vi "Main.vi"(11 "Module Admin":refnum<class "Delacor_lib_QMH_Cloneable Module Admin.lvclass">) -> ()   [LabVIEW 2020, in "DQMH module.lvlib"]
doc: "This template is based off of the Queued Message Handler design pattern and the Queued Message Handler project template that ships with LabVIEW.\n\nThe main difference is that the queue is private to this module and communication between modules is performed via Broadcast and Request events.\n\nRequest events are wrapped in public API methods and are handled in the Event Handling Loop (EHL) of this VI. Any module can register for Broadcast events sent by this module. The EHL generates messages based on user interface actions.\n\nThe Message Handling Loop (MHL) processes messages generated by the EHL, or by other messages. The messages are string values, so new messages can be added easily to the Message Cases case structure in the MHL. Each message cluster can also provide an optional value for Message Data, which is a variant that can be converted to whatever message-specific data is required.\n_____\nBased on Delacor QMH Project Template 5.0.0.82."
uses:
  DQMH module.lvlib
  <vilib>/Delacor/Delacor QMH/Libraries/Cloneable Module Admin_class/Delacor_lib_QMH_Cloneable Module Admin.lvclass
  C:/Program Files (x86)/National Instruments/LabVIEW 2020/vi.lib/Delacor/Delacor QMH/Libraries/Module Admin_class/Delacor_lib_QMH_Module Admin.lvclass
  implementations/Combo box/serial device brand.ctl
  Module Data--cluster.ctl
  <vilib>/Delacor/Delacor QMH/Libraries/Cloneable Module Admin_class/Delacor_lib_QMH_Cloneable Module Admin.lvclass/Delacor_lib_QMH_Cloneable Module Admin.ctl
  Stop Argument--cluster.ctl
  <vilib>/Delacor/Delacor QMH/Libraries/Message Queue_class/Delacor_lib_QMH_Message Queue.lvclass/Delacor_lib_QMH_Message Queue.ctl
  <vilib>/Delacor/Delacor QMH/Libraries/Module Admin_class/Delacor_lib_QMH_Module Admin.lvclass/Delacor_lib_QMH_Module Admin.ctl
  Read ADC Argument--cluster.ctl
  Set Port Status Argument--cluster.ctl
  Get Port Status Argument--cluster.ctl
  Set Pin Argument--cluster.ctl
  Get Pin Status Argument--cluster.ctl
  <vilib>/Utility/miscctls.llb/LVPointTypeDef.ctl
  implementations/Arduino/Arduino.lvclass
  D:/fork/Hal-Proyecto-/Abstracts/Serial Device/Serial Device.lvclass
  Abstracts/Serial Device/Serial Device.lvclass
  implementations/Cypress/Cypress.lvclass
  implementations/Simulado/Simulado.lvclass
  <vilib>/Delacor/Delacor QMH/Libraries/Cloneable Module Admin_class/Delacor_lib_QMH_Get Module ID.vi
  <vilib>/Delacor/Delacor QMH/Libraries/Message Queue_class/Delacor_lib_QMH_Enqueue Message (Single).vi
  <vilib>/Delacor/Delacor QMH/Libraries/Module Admin_class/Delacor_lib_QMH_Get External Launch.vi
  <vilib>/Utility/error.llb/Error Cluster From Error Code.vi
  <vilib>/ErrorRing/Error Ring.xnode
  <vilib>/Delacor/Delacor QMH/Libraries/Message Queue_class/Delacor_lib_QMH_Message Queue.lvclass
panel:
  in  "Configurar":bool
  in  "VISA resource name":refnum<visa-resource-name>
  in  "Serial Device Brand":T1
  out "Respuesta":string
  in  "CH":dbl
  in  "Read ADC":bool
  in  "Value":string
  in  "Puerto":dbl
  in  "Set port":bool
  out "Port status":bool[](array[boolean])
  in  "Port":dbl
  in  "Get port":bool
  in  "Value":bool
  in  "Pin":dbl
  in  "Port 2":dbl
  in  "Set Pin":bool
  out "error out":errorcluster
  out "Value":bool
  in  "Pin 2":dbl
  in  "Port 3":dbl
  in  "Get pin":bool
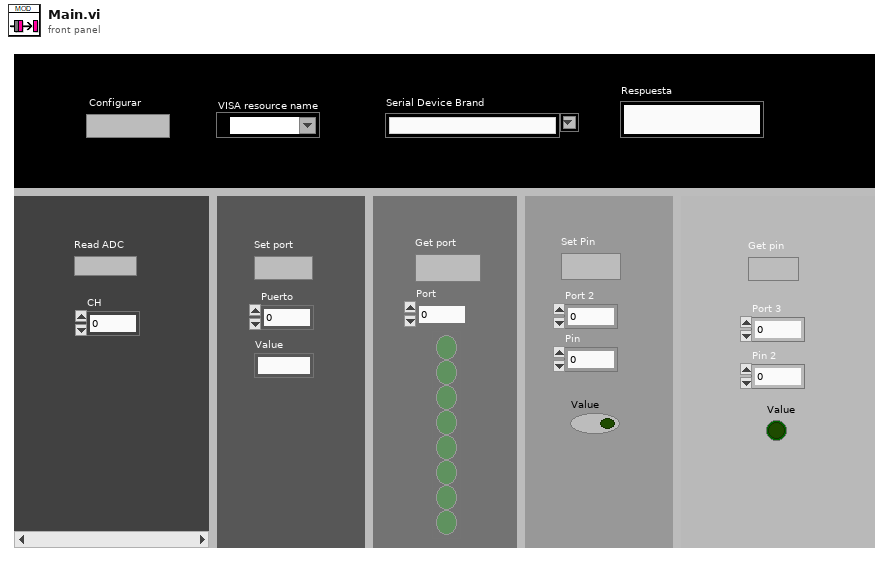
[diagram p1: front panel]
types:
  T1 = typedef "Serial Device.lvclass/serial device brand.ctl" = string
  T2 = typedef "DQMH module.lvlib/Request Events--cluster.ctl" = cluster{"Stop Module":refnum<user-event>, "Show Panel":refnum<user-event>, "Hide Panel":refnum<user-event>, "Show Diagram":refnum<user-event>, "Get Module Execution Status":refnum<user-event>, "Read ADC":refnum<user-event>, "Set Port Status":refnum<user-event>, "Get Port Status":refnum<user-event>, "Set Pin":refnum<user-event>, "Get Pin Status":refnum<user-event>}
  T3 = typedef "DQMH module.lvlib/Module Data--cluster.ctl" = cluster{"Status":string}
  T4 = enum32{"invalid lock state", "Not Locked", "Locked (No Password)", "Password-protected"}
  T5 = typedef "DQMH module.lvlib/Stop Argument--cluster.ctl" = cluster{"Module ID":i32, "Origin":string, "Exit via Stop Module Req?":bool, "Wait for Module to stop?":bool}
  T6 = typedef "DQMH module.lvlib/Read ADC Argument--cluster.ctl" = cluster{"Module ID":i32, "CH ADC":dbl}
  T7 = typedef "DQMH module.lvlib/Set Port Status Argument--cluster.ctl" = cluster{"Module ID":i32, "Puerto":dbl, "Value":string}
  T8 = typedef "DQMH module.lvlib/Get Port Status Argument--cluster.ctl" = cluster{"Module ID":i32, "Port":dbl}
  T9 = typedef "DQMH module.lvlib/Set Pin Argument--cluster.ctl" = cluster{"Module ID":i32, "Port":dbl, "Pin":dbl, "Value":bool}
  T10 = typedef "DQMH module.lvlib/Get Pin Status Argument--cluster.ctl" = cluster{"Module ID":i32, "Port":dbl, "Pin":dbl, "Valor de Pin":bool}
  T11 = enum32{"Invalid", "Standard", "Closed", "Hidden", "Minimized", "Maximized"}
  T12 = typedef "LVPointTypeDef.ctl" = cluster{"Horizontal":i16, "Vertical":i16}
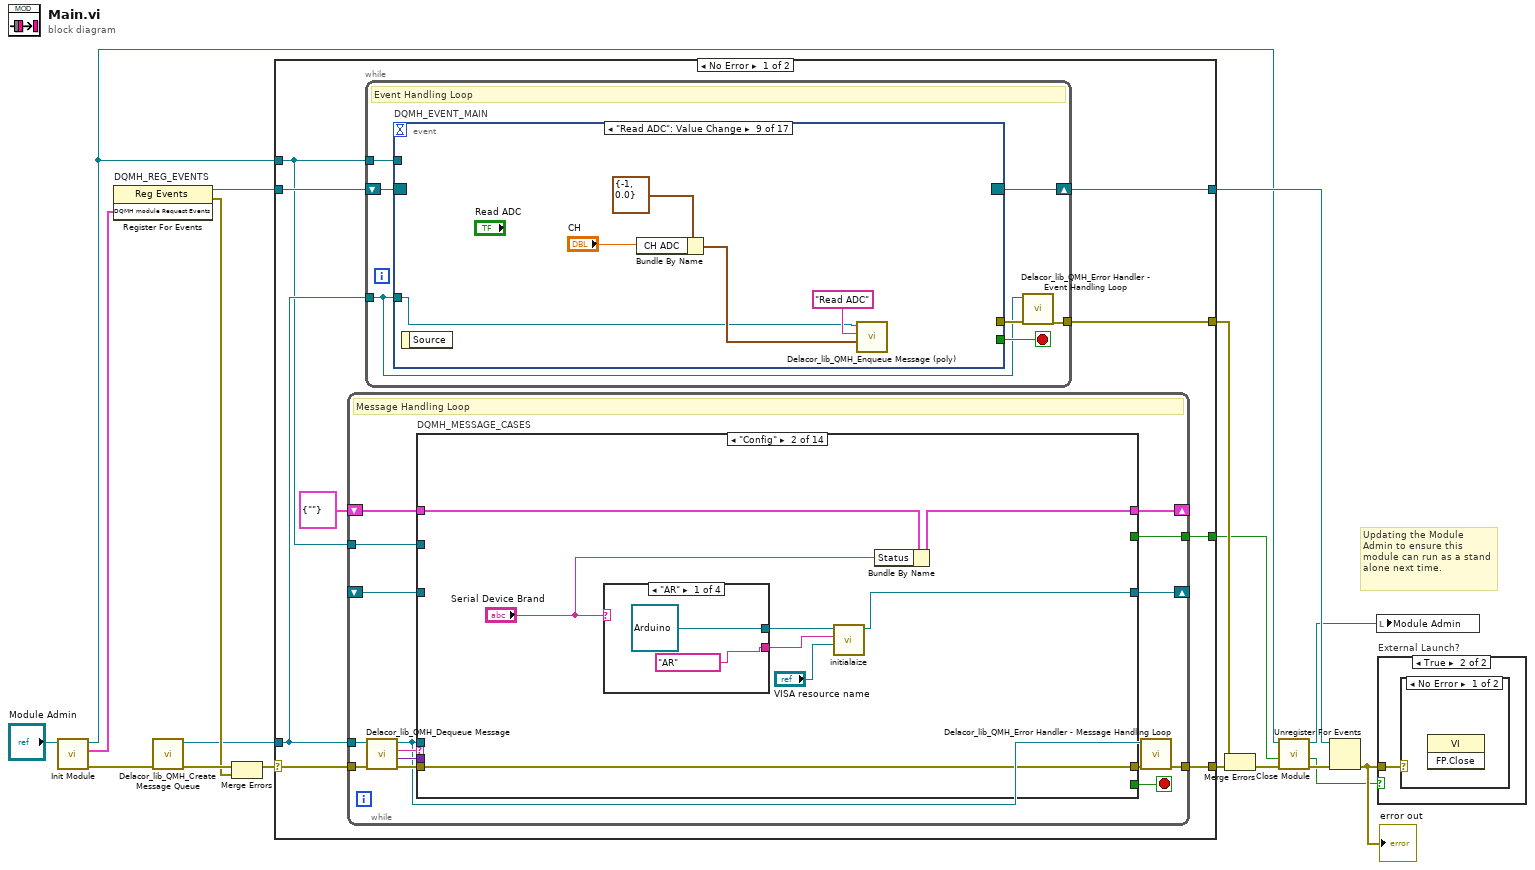
[diagram p0: block diagram]
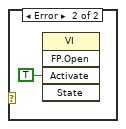
[diagram p3: hidden frame]
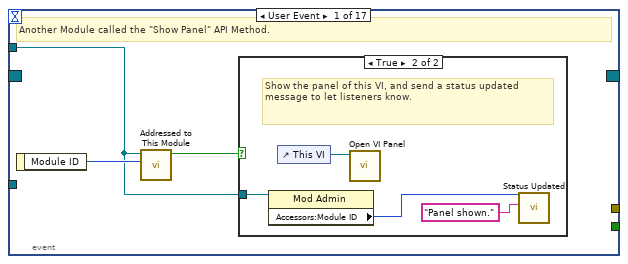
[diagram p4: hidden frame]
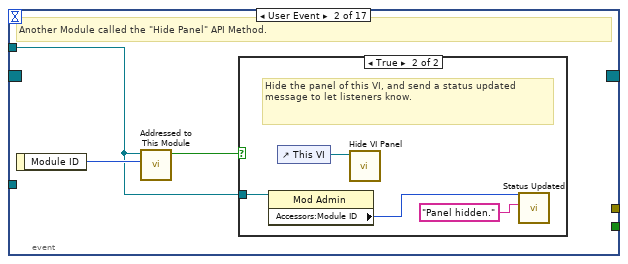
[diagram p6: hidden frame]
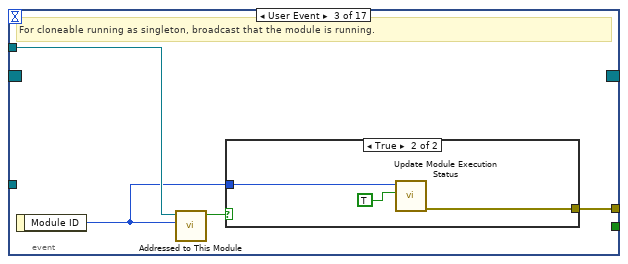
[diagram p8: hidden frame]
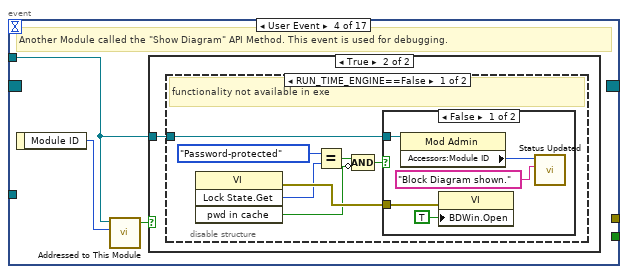
[diagram p10: hidden frame]
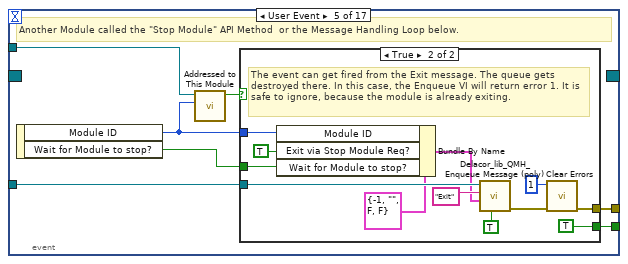
[diagram p14: hidden frame]
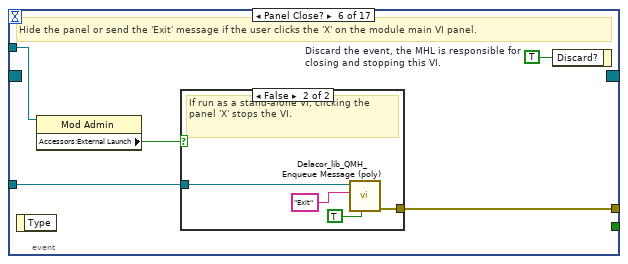
[diagram p16: hidden frame]
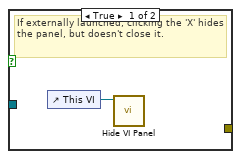
[diagram p17: hidden frame]
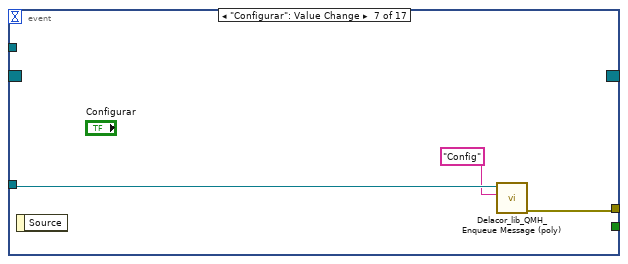
[diagram p18: hidden frame]
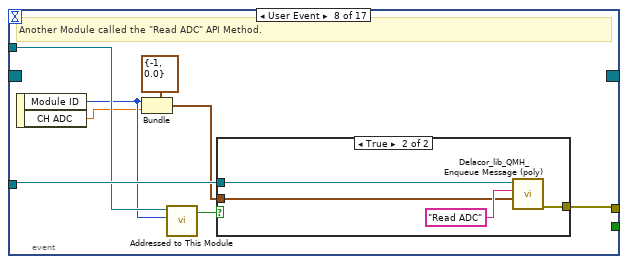
[diagram p19: hidden frame]
diagram:
  # "Updating the Module Admin to ensure this module can run as a stand alone next time."
  n1 = call "Init Module.vi"("Cloneable Module Admin in"="Module Admin") -> ("error out"=w15:errorcluster, "DQMH module Request Events"=w7:T2, "Cloneable Module Admin out"=w4:refnum<class "Delacor_lib_QMH_Cloneable Module Admin.lvclass">)  [unwired: 8 in]
  n2 = register-events "DQMH_REG_EVENTS"(w7) -> (reference out=w8:refnum<event-registration>, error out=w10:errorcluster)  [unwired: 2 in]
  n3 = call <vilib>:"Delacor_lib_QMH_Create Message Queue.vi"("error in (no error)"=w15) -> ("error out"=w12:errorcluster, "Message Queue"=w6:refnum<class "Delacor_lib_QMH_Message Queue.lvclass">)  [unwired: 9 in]
  n4 = Merge Errors(w12, w10) -> (w11:errorcluster)
  n5 = case shown="No Error" w11 {
    selector: w11 -> [w25 w417]
    tunnel: [w27 w416] -> w16
    tunnel: [w24 w424] -> w9
    tunnel: w8 -> [w22 w424]
    tunnel: w6 -> [w21 w415]
    tunnel: [w26 _] -> w17
    tunnel: w4 -> [w20 w420]
    tunnel: [w19 _] -> w2
    frame No Error {
      n6 = while {
        tunnel: w21 -> [w207]
        shift-right: [w211] -> _
        shift-left: T3 {"Status"=""} ("Data Cluster") -> [w212]
        tunnel: w25 -> [w215]
        tunnel: [w213] -> w27
        tunnel: w20 -> [w205]
        tunnel: [w204] -> w19
        shift-right: [w203] -> _
        shift-left: _ -> [w202]
        stop <- w210 stop-if-true
        # "Message Handling Loop"
        n7 = call-dynamic "Delacor_lib_QMH_Dequeue Message.vi"("error in (no error)"=w215, "Message Queue in"=w207) -> ("error out"=w214:errorcluster, "Message Data"=w208:variant, "Message"=w209:string, "Message Queue out"=w206:refnum<class "Delacor_lib_QMH_Message Queue.lvclass">)  [unwired: 6 in]
        n8 = case "DQMH_MESSAGE_CASES" shown="\"Config\"" w209 {
          selector: w209 -> [_ _ _ _ _ _ _ _ _ _ _ _ _ w402]
          tunnel: w206 -> [_ _ _ w256 _ w282 _ w320 _ _ _ w358 w391 _]
          tunnel: w214 -> [w233 w243 w254 w270 w275 w294 w310 w329 w346 w350 w353 w366 w397 w404]
          tunnel: [w231 w243 w254 w258 w276 w285 w300 w318 w334 w349 w353 w362 w394 w405] -> w216
          tunnel: w212 -> [w217 w238 w253 w269 w277 w293 w309 w328 w345 w348 w352 w356 w390 w403]
          tunnel: [w217 w239 w253 w269 w277 w293 w309 w328 w345 w348 w352 w356 w390 w403] -> w211
          tunnel: [_ _ _ _ _ _ _ _ _ _ _ _ w389 _] -> w210
          tunnel: w208 -> [_ _ _ w268 w274 w292 w308 w327 w344 _ _ w361 w387 _]
          tunnel: w205 -> [w220 _ _ _ _ _ _ _ _ _ _ w360 w383 w400]
          tunnel: [_ _ _ _ _ _ _ _ _ _ _ _ w385 _] -> w204
          tunnel: [w218 w236 w252 w255 w271 w280 w303 w321 w339 w347 w351 w354 w380 w398] -> w203
          tunnel: w202 -> [w218 _ w252 w265 w271 w289 w305 w323 w340 w347 w351 w354 w381 w398]
          frame "Initialize" {
            (unwired) T12 {"Horizontal"=0, "Vertical"=0} ("Origin")
            # "Initialize - Any operation that needs to be done before the module can receive messages. Synchronize Caller Events.vi will inform Start Module.vi that the module has launched and is ready to receive messages. Module Did Init.vi will broadcast that the module initialized."
            n9 = call "Synchronize Caller Events.vi"("error in (no error)"=w233, "Module Admin"=w220) -> ("error out"=w232:errorcluster, "Module Admin out"=w219:refnum<class "Delacor_lib_QMH_Cloneable Module Admin.lvclass">)  [unwired: 8 in]
            n10 = property class="Mod Admin"(reference=w219) -> ("Accessors:Module ID"=w222:i32, "Accessors:External Launch"=w221:bool)  [unwired: 1 in, 2 out]
            n11 = call "Module Name--constant.vi"("Module ID"=w222) -> ("Module Name"=w228:string)  [unwired: 10 in]
            n12 = property class="VI"("Front Panel.Title"=w228) -> (reference out=w230:refnum<vi>, error out=w235:errorcluster)  [unwired: 2 in]
            n13 = Select(t=T11."Hidden" ("State"), s=w221, f=T11."Standard" ("State")) -> (s? t:f=w225:T11)
            n14 = invoke class="VI" method="FP.Open"(reference=w230, error in=w235, "State"=w225) -> (reference out=w229:refnum<vi>, error out=w234:errorcluster)  [unwired: 2 in, 3 out]
            n15 = call "Module Name--constant.vi"("Module ID"=w222) -> ("Module Name"=w223:string)  [unwired: 10 in]
            n16 = invoke class="VI" method="FP.Center"(reference=w229, error in=w234) -> ()  [unwired: 1 in, 3 out]
            n17 = call "Module Did Init.vi"("error in (no error)"=w232, "Initialized?"=TRUE, "Origin"=w223, "Module ID"=w222) -> ("error out"=w231:errorcluster)  [unwired: 7 in]
          }
          frame "Config" {
            n18 = case shown="\"AR\"" "Serial Device Brand" {
              tunnel: [refnum<class "Arduino.lvclass"> refnum ("Arduino.lvclass") refnum<class "Serial Device.lvclass"> refnum ("Cypress.lvclass") refnum<class "Cypress.lvclass"> refnum ("Cypress.lvclass") refnum<class "Simulado.lvclass"> refnum ("Simulado.lvclass")] -> w242
              tunnel: [T1 "AR" ("Serial Device Brand 2") T1 "NX" ("Serial Device Brand 2") T1 "CY" ("Serial Device Brand 2") T1 "SD" ("Serial Device Brand 2")] -> w240
              frame "AR" {
              }
              frame "NX" {
              }
              frame "CY" {
              }
              frame "SD", Default {
              }
            }
            n19 = call-dynamic "initialaize.vi"("Visa com port"="VISA resource name", "Serial Device Brand"=w240, "Serial Device in"=w242) -> ("Serial Device out"=w236:refnum<class "Serial Device.lvclass">)  [unwired: 7 in, 1 out]
            n20 = Bundle By Name(cluster=w238, "Status"="Serial Device Brand") -> (w239:T3)
          }
          frame "--- Module Specific ---" {
            # "Separator -- The following cases handle messages specific to this Module."
          }
          frame "Read ADC" {
            n21 = Variant To Data(error in=w270, type=T6 {"Module ID"=-1, "CH ADC"=0.0} ("Read ADC Argument"), Variant=w268) -> (data=w266:T6, error out=w259:errorcluster)
            n22 = Unbundle By Name(w266) -> ("CH ADC"=w263:dbl)
            n23 = call-dynamic "Read ADC.vi"("ADC CH"=w263, "Serial Device in"=w265) -> ("error out"=w262:errorcluster, "Serial Device out"=w264:refnum<class "Serial Device.lvclass">)  [unwired: 8 in]
            n24 = call-dynamic "Read Response ADC.vi"("error in (no error)"=w262, "Serial Device in"=w264) -> ("Respuesta"=w261:string, "Serial Device out"=w255:refnum<class "Serial Device.lvclass">)  [unwired: 7 in, 1 out]
            n25 = call-poly <vilib>:"Delacor_lib_QMH_Enqueue Message (poly).vi"("Message Data"=w261, "Message"="Response", "Message Queue in"=w256) -> ("error out"=w257:errorcluster)  [unwired: 7 in, 1 out]
            n26 = Merge Errors(w257, w259) -> (w258:errorcluster)
          }
          frame "Response" {
            n27 = Variant To Data(error in=w275, type="", Variant=w274) -> (data=→"Respuesta":string, error out=w276:errorcluster)
          }
          frame "Set Port Status" {
            n28 = Variant To Data(error in=w294, type=T7 {"Module ID"=-1, "Puerto"=0.0, "Value"=""} ("Set Port Status Argument"), Variant=w292) -> (data=w290:T7, error out=w286:errorcluster)
            n29 = Unbundle By Name(w290) -> ("Puerto"=w279:dbl, "Value"=w278:string)
            n30 = call-dynamic "Set port.vi"("Value"=w278, "Puerto"=w279, "Serial Device in"=w289) -> ("error out"=w287:errorcluster, "Serial Device out"=w288:refnum<class "Serial Device.lvclass">)  [unwired: 7 in]
            n31 = call-dynamic "Read Response ADC.vi"("error in (no error)"=w287, "Serial Device in"=w288) -> ("Respuesta"=w281:string, "Serial Device out"=w280:refnum<class "Serial Device.lvclass">)  [unwired: 7 in, 1 out]
            n32 = call-poly <vilib>:"Delacor_lib_QMH_Enqueue Message (poly).vi"("Message Data"=w281, "Message"="Response", "Message Queue in"=w282) -> ("error out"=w284:errorcluster)  [unwired: 7 in, 1 out]
            n33 = Merge Errors(w284, w286) -> (w285:errorcluster)
          }
          frame "Get Port Status" {
            n34 = Variant To Data(error in=w310, type=T8 {"Module ID"=-1, "Port"=0.0} ("Get Port Status Argument"), Variant=w308) -> (data=w306:T8, error out=w299:errorcluster)
            n35 = Unbundle By Name(w306) -> ("Port"=w302:dbl)
            n36 = call-dynamic "Get port Status.vi"("Puerto"=w302, "Serial Device in"=w305) -> ("error out"=w298:errorcluster, "Serial Device out"=w304:refnum<class "Serial Device.lvclass">)  [unwired: 8 in]
            n37 = call-dynamic "Get status Response.vi"("error in (no error)"=w298, "Serial Device in"=w304) -> ("error out"=w297:errorcluster, "Response"=w301:string, "Serial Device out"=w303:refnum<class "Serial Device.lvclass">)  [unwired: 7 in]
            n38 = Hexadecimal String To Number(string=w301) -> (number=w296:u32)  [unwired: 2 in, 1 out]
            n39 = Number To Boolean Array(number=w296) -> (Boolean array=→"Port status":bool[])
            n40 = Merge Errors(w297, w299) -> (w300:errorcluster)
          }
          frame "Set Pin" {
            n41 = Variant To Data(error in=w329, type=T9 {"Module ID"=-1, "Port"=0.0, "Pin"=0.0, "Value"=FALSE} ("Set Pin Argument"), Variant=w327) -> (data=w325:T9, error out=w319:errorcluster)
            n42 = Unbundle By Name(w325) -> ("Port"=w314:dbl, "Pin"=w313:dbl, "Value"=w312:bool)
            n43 = call-dynamic "Set pin status.vi"("Value"=w312, "Pin"=w313, "Port"=w314, "Serial Device in"=w323) -> ("error out"=w324:errorcluster, "Serial Device out"=w322:refnum<class "Serial Device.lvclass">)  [unwired: 6 in]
            n44 = call-dynamic "Read Response ADC.vi"("error in (no error)"=w324, "Serial Device in"=w322) -> ("error out"=w315:errorcluster, "Respuesta"=w311:string, "Serial Device out"=w321:refnum<class "Serial Device.lvclass">)  [unwired: 7 in]
            n45 = call-poly <vilib>:"Delacor_lib_QMH_Enqueue Message (poly).vi"("error in (no error)"=w315, "Message Data"=w311, "Message"="Response", "Message Queue in"=w320) -> ("error out"=w317:errorcluster)  [unwired: 6 in, 1 out]
            n46 = Merge Errors(w317, w319) -> (w318:errorcluster)
          }
          frame "Get Pin Status" {
            n47 = Variant To Data(error in=w346, type=T10 {"Module ID"=-1, "Port"=0.0, "Pin"=0.0, "Valor de Pin"=FALSE} ("Get Pin Status Argument"), Variant=w344) -> (data=w342:T10, error out=w335:errorcluster)
            n48 = Unbundle By Name(w342) -> ("Port"=w337:dbl, "Pin"=w336:dbl)
            n49 = call-dynamic "Get pin Status.vi"("Pin 2"=w336, "Puerto"=w337, "Serial Device in"=w340) -> ("error out"=w338:errorcluster, "Serial Device out"=w341:refnum<class "Serial Device.lvclass">)  [unwired: 7 in]
            n50 = call-dynamic "Get pin Status Response.vi"("error in (no error)"=w338, "Serial Device in"=w341) -> ("Value"=w333:string, "Serial Device out"=w339:refnum<class "Serial Device.lvclass">)  [unwired: 7 in, 1 out]
            n51 = Hexadecimal String To Number(string=w333) -> (number=w332:u32)  [unwired: 2 in, 1 out]
            n52 = Equal To 0?(x=w332) -> (x = 0?=w331:bool)
            n53 = Not(x=w331) -> (.not. x?=→"Value":bool)
            n54 = Merge Errors(w335) -> (w334:errorcluster)
          }
          frame "---Copy This Frame---" {
            # "Duplicate this frame when creating new messages.  Change this comment in the duplicated frame to describe this message."
            n55 = Merge Errors(w350) -> (w349:errorcluster)
          }
          frame "--- Exit and Error Handling---" {
            # "Separator - the following cases handle errors and exit messages."
          }
          frame "Error" {
            # "Error - Check the error message data and respond accordingly. This message is sent by the \"Error Handler\" VIs at the end of each loop in this application."
            n56 = property class="Mod Admin"(reference=w360) -> ("Accessors:External Launch"=w359:bool, "Accessors:Module ID"=w357:i32)  [unwired: 1 in, 2 out]
            n57 = Variant To Data(error in=w366, type=errorcluster {"status"=FALSE, "code"=0, "source"=""} ("error constant"), Variant=w361) -> (data=w367:errorcluster, error out=w364:errorcluster)
            n58 = Unbundle By Name(w356) -> ("Status"=w355:string)
            n59 = call "Module Name--constant.vi"("Module ID"=w357) -> ()  [unwired: 10 in, 1 out]
            n60 = case shown="True" w359 {
              tunnel: [w372 w374] -> w363
              tunnel: w358 -> [w370 w376]
              tunnel: w367 -> [w371 _]
              tunnel: w355 -> [_ w379]
              frame False {
                n61 = call <vilib>:"Simple Error Handler.vi"("error in (no error)"=w371) -> ()  [unwired: 4 in, 5 out]
                n62 = call-poly <vilib>:"Delacor_lib_QMH_Enqueue Message (poly).vi"("Priority Message? (F)"=TRUE, "Message"="Exit", "Message Queue in"=w370) -> ("error out"=w372:errorcluster)  [unwired: 7 in, 1 out]
              }
              frame True {
                n63 = Concatenate Strings("Micro desconectado" ("string"), w379) -> (w377:string)
                n64 = call-poly <vilib>:"Delacor_lib_QMH_Enqueue Message (poly).vi"("Priority Message? (F)"=TRUE, "Message"="EXIT", "Message Queue in"=w376) -> ("error out"=w374:errorcluster)  [unwired: 7 in, 1 out]
                n65 = One Button Dialog(message=w377) -> ()  [unwired: 1 in, 1 out]
              }
            }
            n66 = call "Error Reported.vi"("Additional Information"=w355, "Error"=w367, "Module ID"=w357) -> ()  [unwired: 8 in, 1 out]
            n67 = Merge Errors(w364, w363) -> (w362:errorcluster)
            n68 = local write "error out"(w362) -> ()
          }
          frame "Exit" {
            w388 = 91  # 91: not all Exit messages will have an argument
            w389 = TRUE  # Stop the VI
            # "Release the message queue reference"
            # "Exit - Exit the application."
            n69 = Variant To Data(error in=w397, type=T5 {"Module ID"=-1, "Origin"="", "Exit via Stop Module Req?"=FALSE, "Wait for Module to stop?"=FALSE} ("Stop Argument"), Variant=w387) -> (data=w384:T5, error out=w392:errorcluster)
            n70 = call <vilib>:"Clear Errors.vi"("error in (no error)"=w392, "specific error code to clear (0: all)"=w388) -> ("error out"=w396:errorcluster)  [unwired: 4 in, 1 out]
            n71 = call-dynamic "close visa.vi"("Serial Device in"=w381) -> ("Serial Device out"=w380:refnum<class "Serial Device.lvclass">)  [unwired: 9 in, 1 out]
            n72 = control-ref of="This VI"() -> (w382:refnum<vi>)
            n73 = call-dynamic "Delacor_lib_QMH_Release Message Queue.vi"("error in (no error)"=w396, "Message Queue"=w391) -> ("error out"=w395:errorcluster)  [unwired: 9 in]
            n74 = call "Handle Exit.vi"("Stop Argument"=w384, "Module Admin in"=w383, "VI reference"=w382) -> ("error out"=w393:errorcluster, "Wait for Stop?"=w385:bool)  [unwired: 7 in]
            n75 = Merge Errors(w395, w393) -> (w394:errorcluster)
          }
          frame Default {
            # "'Default' case only runs if there is a message that isn't defined in any of the other cases.  Output a programming error."
            n76 = property class="Mod Admin"(reference=w400) -> ("Accessors:Module ID"=w399:i32)  [unwired: 1 in, 2 out]
            n77 = call "Module Name--constant.vi"("Module ID"=w399) -> ("Module Name"=w401:string)  [unwired: 10 in]
            n78 = xnode "Error Ring"("parameter 0"=w402, "parameter 1"=w401) -> ("error out"=w406:errorcluster)
            n79 = Merge Errors(w404, w406) -> (w405:errorcluster)
          }
        }
        n80 = call-dynamic "Delacor_lib_QMH_Error Handler - Message Handling Loop.vi"("error in (no error)"=w216, "Message Queue in"=w206) -> ("dup error in"=w213:errorcluster)  [unwired: 8 in, 1 out]
      }
      n81 = while {
        tunnel: w21 -> [w28]
        shift-right: [w31] -> w24
        shift-left: w22 -> [w32]
        tunnel: [w33] -> w26
        tunnel: w20 -> [w29]
        stop <- w30 stop-if-true
        # "Event Handling Loop"
        n82 = event "DQMH_EVENT_MAIN" shown="[8] \"Read ADC\": Value Change" {
          selector: w32 -> [_ _ _ _ _ _ _ _ _ _ _ _ _ _ _ _ _]
          dyn-events: [_ _ _ _ _ _ _ _ _ _ _ _ _ _ _ _ _] -> w31
          timeout: _ -> [_ _ _ _ _ _ _ _ _ _ _ _ _ _ _ _ _]
          tunnel: [_ _ _ _ w74 _ _ _ _ _ _ _ _ _ _ _ _] -> w30
          tunnel: w28 -> [_ _ _ _ w77 w92 w103 w111 w116 w129 w134 w148 w155 w168 w180 w190 w201]
          tunnel: [_ _ w52 _ w78 w95 w102 w104 _ w121 w135 w141 w156 w159 w179 w181 w200] -> w34
          tunnel: w29 -> [w35 w42 w50 w56 w76 w93 _ w109 _ w127 _ w146 _ w166 _ w188 _]
          event User Event {
            # "Another Module called the \"Show Panel\" API Method."
            n83 = event-data() -> ("Module ID"=w36:i32)  [unwired: 1 in]
            n84 = call "Addressed to This Module.vi"("Module ID from Argument"=w36, "Module Admin"=w35) -> ("Addressed to this instance?"=w37:bool)  [unwired: 8 in, 1 out]
            n85 = case shown="True" w37 {
              tunnel: w35 -> [_ w39]
              frame False {
              }
              frame True {
                # "Show the panel of this VI, and send a status updated message to let listeners know."
                n86 = property class="Mod Admin"(reference=w39) -> ("Accessors:Module ID"=w38:i32)  [unwired: 1 in, 2 out]
                n87 = control-ref of="This VI"() -> (w41:refnum<vi>)
                n88 = call "Open VI Panel.vi"("VI"=w41) -> ()  [unwired: 10 in, 1 out]
                n89 = call "Status Updated.vi"("Status"="Panel shown." ("format string"), "Module ID"=w38) -> ()  [unwired: 9 in, 1 out]
              }
            }
          }
          event User Event {
            # "Another Module called the \"Hide Panel\" API Method."
            n90 = event-data() -> ("Module ID"=w43:i32)  [unwired: 1 in]
            n91 = call "Addressed to This Module.vi"("Module ID from Argument"=w43, "Module Admin"=w42) -> ("Addressed to this instance?"=w44:bool)  [unwired: 8 in, 1 out]
            n92 = case shown="True" w44 {
              tunnel: w42 -> [_ w46]
              frame False {
              }
              frame True {
                # "Hide the panel of this VI, and send a status updated message to let listeners know."
                n93 = property class="Mod Admin"(reference=w46) -> ("Accessors:Module ID"=w45:i32)  [unwired: 1 in, 2 out]
                n94 = control-ref of="This VI"() -> (w48:refnum<vi>)
                n95 = call "Hide VI Panel.vi"("VI"=w48) -> ()  [unwired: 10 in, 1 out]
                n96 = call "Status Updated.vi"("Status"="Panel hidden." ("format string"), "Module ID"=w45) -> ()  [unwired: 9 in, 1 out]
              }
            }
          }
          event User Event {
            # "For cloneable running as singleton, broadcast that the module is running."
            n97 = event-data() -> ("Module ID"=w49:i32)  [unwired: 1 in]
            n98 = call "Addressed to This Module.vi"("Module ID from Argument"=w49, "Module Admin"=w50) -> ("Addressed to this instance?"=w51:bool)  [unwired: 8 in, 1 out]
            n99 = case shown="True" w51 {
              tunnel: [_ w55] -> w52
              tunnel: w49 -> [_ w54]
              frame False {
              }
              frame True {
                n100 = call "Update Module Execution Status.vi"("Running?"=TRUE, "Module ID"=w54) -> ("error out"=w55:errorcluster)  [unwired: 9 in]
              }
            }
          }
          event User Event {
            # "Another Module called the \"Show Diagram\" API Method. This event is used for debugging."
            n101 = event-data() -> ("Module ID"=w57:i32)  [unwired: 1 in]
            n102 = call "Addressed to This Module.vi"("Module ID from Argument"=w57, "Module Admin"=w56) -> ("Addressed to this instance?"=w58:bool)  [unwired: 8 in, 1 out]
            n103 = case shown="True" w58 {
              tunnel: w56 -> [_ w59]
              frame False {
              }
              frame True {
                n104 = disable-structure shown="RUN_TIME_ENGINE==False" {
                  disable-tunnel: w59 -> [w60 _]
                  frame condition #0 (active) {
                    # "functionality not available in exe"
                    n105 = invoke class="VI" method="Lock State.Get"() -> (error out=w66:errorcluster, "Get Lock State"=w65:T4, "pwd in cache"=w62:bool)  [unwired: 4 in, 1 out]
                    n106 = Equal?(x=T4."Password-protected", y=w65) -> (x = y?=w63:bool)
                    n107 = Compound Arithmetic op=AND(w63, invert w62) -> (w61:bool)
                    n108 = case shown="False" w61 {
                      tunnel: w66 -> [w71 _]
                      tunnel: w60 -> [w68 _]
                      frame False {
                        n109 = property class="Mod Admin"(reference=w68) -> ("Accessors:Module ID"=w67:i32)  [unwired: 1 in, 2 out]
                        n110 = property class="VI"(error in=w71, "BDWin.Open"=TRUE ("Block Diagram Window:Open")) -> ()  [unwired: 1 in, 2 out]
                        n111 = call "Status Updated.vi"("Status"="Block Diagram shown." ("format string"), "Module ID"=w67) -> ()  [unwired: 9 in, 1 out]
                      }
                      frame True {
                        # "Password-protected VI, and the password is not in the cache. Do not show the diagram."
                      }
                    }
                  }
                  frame condition #1 {
                  }
                }
              }
            }
          }
          event User Event {
            # "Another Module called the \"Stop Module\" API Method  or the Message Handling Loop below."
            n112 = event-data() -> ("Module ID"=w72:i32, "Wait for Module to stop?"=w73:bool)  [unwired: 1 in]
            n113 = call "Addressed to This Module.vi"("Module ID from Argument"=w72, "Module Admin"=w76) -> ("Addressed to this instance?"=w75:bool)  [unwired: 8 in, 1 out]
            n114 = case shown="True" w75 {
              tunnel: [_ w89] -> w78
              tunnel: w77 -> [_ w85]
              tunnel: [_ TRUE] -> w74
              tunnel: w73 -> [_ w80]
              tunnel: w72 -> [_ w82]
              frame False {
              }
              frame True {
                # "The event can get fired from the Exit message. The queue gets destroyed there. In this case, the Enqueue VI will return error 1. It is safe to ignore, because the module is already exiting."
                n115 = Bundle By Name(cluster=T5 {"Module ID"=-1, "Origin"="", "Exit via Stop Module Req?"=FALSE, "Wait for Module to stop?"=FALSE} ("Stop Argument"), "Module ID"=w82, "Exit via Stop Module Req?"=TRUE, "Wait for Module to stop?"=w80) -> (w79:T5)
                n116 = call-poly <vilib>:"Delacor_lib_QMH_Enqueue Message (poly).vi"("Priority Message? (F)"=TRUE, "Message Data"=w79, "Message"="Exit", "Message Queue in"=w85) -> ("error out"=w90:errorcluster)  [unwired: 6 in, 1 out]
                n117 = call <vilib>:"Clear Errors.vi"("error in (no error)"=w90, "specific error code to clear (0: all)"=1) -> ("error out"=w89:errorcluster)  [unwired: 4 in, 1 out]
              }
            }
          }
          event Panel Close? {
            w94 = TRUE  # Discard the event, the MHL is responsible for closing and stopping this VI.
            # "Hide the panel or send the 'Exit' message if the user clicks the 'X' on the module main VI panel."
            n118 = event-data() -> ()  [unwired: 1 in, 1 out]
            n119 = property class="Mod Admin"(reference=w93) -> ("Accessors:External Launch"=w91:bool)  [unwired: 1 in, 2 out]
            n120 = case shown="False" w91 {
              tunnel: w92 -> [_ w99]
              tunnel: [_ w100] -> w95
              frame True {
                # "If externally launched, clicking the 'X' hides the panel, but doesn't close it."
                n121 = control-ref of="This VI"() -> (w96:refnum<vi>)
                n122 = call "Hide VI Panel.vi"("VI"=w96) -> ()  [unwired: 10 in, 1 out]
              }
              frame False {
                # "If run as a stand-alone VI, clicking the panel 'X' stops the VI."
                n123 = call-poly <vilib>:"Delacor_lib_QMH_Enqueue Message (poly).vi"("Priority Message? (F)"=TRUE, "Message"="Exit", "Message Queue in"=w99) -> ("error out"=w100:errorcluster)  [unwired: 7 in, 1 out]
              }
            }
            n124 = event-data("Discard?"=w94) -> ()  [unwired: 1 in, 1 out]
          }
          event "Configurar": Value Change {
            n125 = event-data() -> ()  [unwired: 1 in, 1 out]
            n126 = call-poly <vilib>:"Delacor_lib_QMH_Enqueue Message (poly).vi"("Message"="Config", "Message Queue in"=w103) -> ("error out"=w102:errorcluster)  [unwired: 8 in, 1 out]
          }
          event User Event {
            # "Another Module called the \"Read ADC\" API Method."
            n127 = event-data() -> ("Module ID"=w106:i32, "CH ADC"=w105:dbl)  [unwired: 1 in]
            n128 = Bundle(cluster=T6 {"Module ID"=-1, "CH ADC"=0.0} ("Read ADC Argument"), "Module ID"=w106, "CH ADC"=w105) -> (w107:T6)
            n129 = call "Addressed to This Module.vi"("Module ID from Argument"=w106, "Module Admin"=w109) -> ("Addressed to this instance?"=w110:bool)  [unwired: 8 in, 1 out]
            n130 = case shown="True" w110 {
              tunnel: w111 -> [_ w115]
              tunnel: w107 -> [_ w113]
              tunnel: [_ w112] -> w104
              frame False {
              }
              frame True {
                n131 = call-poly <vilib>:"Delacor_lib_QMH_Enqueue Message (poly).vi"("Message Data"=w113, "Message"="Read ADC", "Message Queue in"=w115) -> ("error out"=w112:errorcluster)  [unwired: 7 in, 1 out]
              }
            }
          }
          event "Read ADC": Value Change {
            n132 = event-data() -> ()  [unwired: 1 in, 1 out]
            n133 = Bundle By Name(cluster=T6 {"Module ID"=-1, "CH ADC"=0.0} ("Read ADC Argument"), "CH ADC"="CH") -> (w118:T6)
            n134 = call-poly <vilib>:"Delacor_lib_QMH_Enqueue Message (poly).vi"("Message Data"=w118, "Message"="Read ADC", "Message Queue in"=w116) -> ()  [unwired: 7 in, 2 out]
          }
          event User Event {
            # "Another Module called the \"Set Port Status\" API Method."
            n135 = event-data() -> ("Module ID"=w124:i32, "Puerto"=w123:dbl, "Value"=w122:string)  [unwired: 1 in]
            n136 = Bundle(cluster=T7 {"Module ID"=-1, "Puerto"=0.0, "Value"=""} ("Set Port Status Argument"), "Module ID"=w124, "Puerto"=w123, "Value"=w122) -> (w125:T7)
            n137 = call "Addressed to This Module.vi"("Module ID from Argument"=w124, "Module Admin"=w127) -> ("Addressed to this instance?"=w128:bool)  [unwired: 8 in, 1 out]
            n138 = case shown="True" w128 {
              tunnel: w129 -> [_ w133]
              tunnel: w125 -> [_ w131]
              tunnel: [_ w130] -> w121
              frame False {
              }
              frame True {
                n139 = call-poly <vilib>:"Delacor_lib_QMH_Enqueue Message (poly).vi"("Message Data"=w131, "Message"="Set Port Status", "Message Queue in"=w133) -> ("error out"=w130:errorcluster)  [unwired: 7 in, 1 out]
              }
            }
          }
          event "Set port": Value Change {
            n140 = event-data() -> ()  [unwired: 1 in, 1 out]
            n141 = Bundle By Name(cluster=T7 {"Module ID"=-1, "Puerto"=0.0, "Value"=""} ("Set Port Status Argument"), "Puerto"="Puerto", "Value"="Value") -> (w140:T7)
            n142 = call-poly <vilib>:"Delacor_lib_QMH_Enqueue Message (poly).vi"("Message Data"=w140, "Message"="Set Port Status", "Message Queue in"=w134) -> ("error out"=w135:errorcluster)  [unwired: 7 in, 1 out]
          }
          event User Event {
            # "Another Module called the \"Get Port Status\" API Method."
            n143 = event-data() -> ("Module ID"=w143:i32, "Port"=w142:dbl)  [unwired: 1 in]
            n144 = Bundle(cluster=T8 {"Module ID"=-1, "Port"=0.0} ("Get Port Status Argument"), "Module ID"=w143, "Port"=w142) -> (w144:T8)
            n145 = call "Addressed to This Module.vi"("Module ID from Argument"=w143, "Module Admin"=w146) -> ("Addressed to this instance?"=w147:bool)  [unwired: 8 in, 1 out]
            n146 = case shown="True" w147 {
              tunnel: w148 -> [_ w152]
              tunnel: w144 -> [_ w150]
              tunnel: [_ w149] -> w141
              frame False {
              }
              frame True {
                n147 = call-poly <vilib>:"Delacor_lib_QMH_Enqueue Message (poly).vi"("Message Data"=w150, "Message"="Get Port Status", "Message Queue in"=w152) -> ("error out"=w149:errorcluster)  [unwired: 7 in, 1 out]
              }
            }
          }
          event "Get port": Value Change {
            n148 = event-data() -> ()  [unwired: 1 in, 1 out]
            n149 = Bundle By Name(cluster=T8 {"Module ID"=-1, "Port"=0.0} ("Get Port Status Argument"), "Port"="Port") -> (w153:T8)
            n150 = call-poly <vilib>:"Delacor_lib_QMH_Enqueue Message (poly).vi"("Message Data"=w153, "Message"="Get Port Status", "Message Queue in"=w155) -> ("error out"=w156:errorcluster)  [unwired: 7 in, 1 out]
          }
          event User Event {
            # "Another Module called the \"Set Pin\" API Method."
            n151 = event-data() -> ("Module ID"=w163:i32, "Port"=w162:dbl, "Pin"=w161:dbl, "Value"=w160:bool)  [unwired: 1 in]
            n152 = Bundle(cluster=T9 {"Module ID"=-1, "Port"=0.0, "Pin"=0.0, "Value"=FALSE} ("Set Pin Argument"), "Module ID"=w163, "Port"=w162, "Pin"=w161, "Value"=w160) -> (w164:T9)
            n153 = call "Addressed to This Module.vi"("Module ID from Argument"=w163, "Module Admin"=w166) -> ("Addressed to this instance?"=w167:bool)  [unwired: 8 in, 1 out]
            n154 = case shown="True" w167 {
              tunnel: w168 -> [_ w172]
              tunnel: w164 -> [_ w170]
              tunnel: [_ w169] -> w159
              frame False {
              }
              frame True {
                n155 = call-poly <vilib>:"Delacor_lib_QMH_Enqueue Message (poly).vi"("Message Data"=w170, "Message"="Set Pin", "Message Queue in"=w172) -> ("error out"=w169:errorcluster)  [unwired: 7 in, 1 out]
              }
            }
          }
          event "Set Pin": Value Change {
            n156 = event-data() -> ()  [unwired: 1 in, 1 out]
            n157 = Bundle By Name(cluster=T9 {"Module ID"=-1, "Port"=0.0, "Pin"=0.0, "Value"=FALSE} ("Set Pin Argument"), "Port"="Port 2", "Pin"="Pin", "Value"="Value") -> (w176:T9)
            n158 = call-poly <vilib>:"Delacor_lib_QMH_Enqueue Message (poly).vi"("Message Data"=w176, "Message"="Set Pin", "Message Queue in"=w180) -> ("error out"=w179:errorcluster)  [unwired: 7 in, 1 out]
          }
          event User Event {
            # "Another Module called the \"Get Pin Status\" API Method."
            n159 = event-data() -> ("Module ID"=w185:i32, "Port"=w184:dbl, "Pin"=w183:dbl, "Valor de Pin"=w182:bool)  [unwired: 1 in]
            n160 = Bundle(cluster=T10 {"Module ID"=-1, "Port"=0.0, "Pin"=0.0, "Valor de Pin"=FALSE} ("Get Pin Status Argument"), "Module ID"=w185, "Port"=w184, "Pin"=w183, "Valor de Pin"=w182) -> (w186:T10)
            n161 = call "Addressed to This Module.vi"("Module ID from Argument"=w185, "Module Admin"=w188) -> ("Addressed to this instance?"=w189:bool)  [unwired: 8 in, 1 out]
            n162 = case shown="True" w189 {
              tunnel: w190 -> [_ w194]
              tunnel: w186 -> [_ w192]
              tunnel: [_ w191] -> w181
              frame False {
              }
              frame True {
                n163 = call-poly <vilib>:"Delacor_lib_QMH_Enqueue Message (poly).vi"("Message Data"=w192, "Message"="Get Pin Status", "Message Queue in"=w194) -> ("error out"=w191:errorcluster)  [unwired: 7 in, 1 out]
              }
            }
          }
          event "Get pin": Value Change {
            n164 = event-data() -> ()  [unwired: 1 in, 1 out]
            n165 = Bundle By Name(cluster=T10 {"Module ID"=-1, "Port"=0.0, "Pin"=0.0, "Valor de Pin"=FALSE} ("Get Pin Status Argument"), "Port"="Port 3", "Pin"="Pin 2") -> (w195:T10)
            n166 = call-poly <vilib>:"Delacor_lib_QMH_Enqueue Message (poly).vi"("Message Data"=w195, "Message"="Get Pin Status", "Message Queue in"=w201) -> ("error out"=w200:errorcluster)  [unwired: 7 in, 1 out]
          }
        }
        n167 = call-dynamic "Delacor_lib_QMH_Error Handler - Event Handling Loop.vi"("error in (no error)"=w34, "Message Queue in"=w28) -> ("dup error in"=w33:errorcluster)  [unwired: 8 in, 1 out]
      }
    }
    frame Error {
      n168 = call "Synchronize Caller Events.vi"("Module Admin"=w420) -> ("Module Admin out"=w419:refnum<class "Delacor_lib_QMH_Cloneable Module Admin.lvclass">)  [unwired: 9 in, 1 out]
      n169 = property class="Mod Admin"(reference=w419) -> ("Accessors:Module ID"=w418:i32)  [unwired: 1 in, 2 out]
      n170 = call-dynamic "Delacor_lib_QMH_Release Message Queue.vi"("error in (no error)"=w417, "Message Queue"=w415) -> ("error out"=w416:errorcluster)  [unwired: 9 in]
      n171 = call "Module Name--constant.vi"("Module ID"=w418) -> ("Module Name"=w423:string)  [unwired: 10 in]
      n172 = Format Into String(format string="An error occurred during initialization. %s is no longer running.", w423) -> (resulting string=w421:string)  [unwired: 2 in, 1 out]
      n173 = call "Error Reported.vi"("Additional Information"=w421, "Error"=w416, "Module ID"=w418) -> ()  [unwired: 8 in, 1 out]
    }
  }
  n174 = Merge Errors(w17, w16) -> (w18:errorcluster)
  n175 = call "Close Module.vi"("error in"=w18, "Wait for stop?"=w2, "Module Admin in"=w4) -> ("error out"=w14:errorcluster, "External Launch"=w1:bool, "Module Admin out"=w3:refnum<class "Delacor_lib_QMH_Cloneable Module Admin.lvclass">)  [unwired: 6 in]
  n176 = Unregister For Events(event registration refnum=w9, error in=w14) -> (error out=w13:errorcluster)
  "error out" <- w13
  n177 = local write "Module Admin"(w3) -> ()
  n178 = case "External Launch?" shown="True" w1 {
    tunnel: w13 -> [_ w425]
    frame False {
    }
    frame True {
      n179 = case shown="No Error" w425 {
        frame No Error {
          n180 = invoke class="VI" method="FP.Close"() -> ()  [unwired: 3 in, 3 out]
        }
        frame Error {
          n181 = invoke class="VI" method="FP.Open"("Activate"=TRUE ("Activate?")) -> ()  [unwired: 4 in, 5 out]
        }
      }
    }
  }
